vi "u16_to_u8.vi"(1 "数值":u16) -> (0 "无符号8位整型":u8)   [LabVIEW 2018]
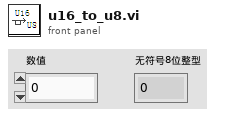
[diagram p1: front panel]
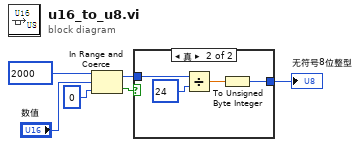
[diagram p0: block diagram]
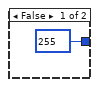
[diagram p2: hidden frame]
diagram:
  n1 = In Range and Coerce(upper limit=u16 2000 ("上限"), x="数值", lower limit=u16 0 ("下限")) -> (coerced(x)=w1:u16, In Range?=w3:bool)
  n2 = case shown="真" w3 {
    tunnel: [u8 255 w8] -> w2
    tunnel: w1 -> [_ w10]
    frame False {
    }
    frame True {
      n3 = Divide(x=w10, y=u16 24) -> (x/y=w11:dbl)
      n4 = To Unsigned Byte Integer(number=w11) -> (unsigned 8bit integer=w8:u8)
    }
  }
  "无符号8位整型" <- w2
